vi "Command.vi"(7 "Cryo Idx":i32, 8 "error in (no error)":errorcluster, 9 "Options":string, 10 "Command":T1 items=["STATUS", "COOLER", "E", "ERROR", "KD", "KI", "KP", "LOGIN", "LOGOUT", "MODE", "P", "PWOUT", "SENSOR", "TC", "TEMP RJ", "TTARGET", "VERSION"], 11 "CryoCoolerAVC in":refnum<class "CryoCoolerAVC.lvclass">) -> (0 "error out":errorcluster, 2 "Response":string[](array[string]), 3 "CryoCoolerAVC out":refnum<class "CryoCoolerAVC.lvclass">)   [LabVIEW 2024, in "CryoCoolerAVC.lvclass"]
uses:
  CryoCoolerAVC.lvclass
  CryoCoolerAVC Command enum.ctl
  CryoCoolerAVC.lvclass/CryoCoolerAVC.ctl
  Cryo Cooler.lvclass
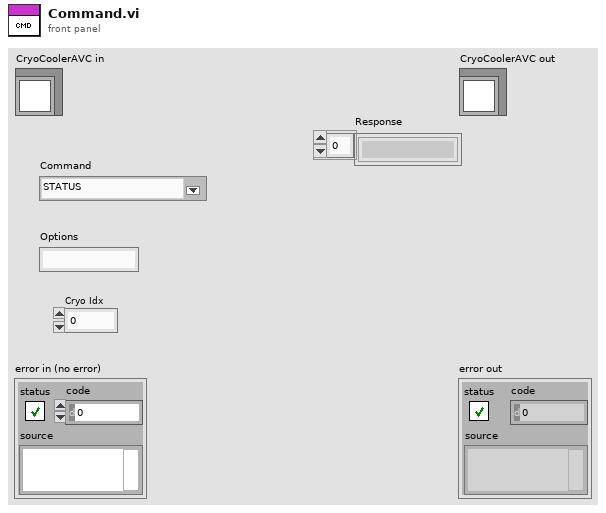
[diagram p1: front panel]
types:
  T1 = typedef "CryoCoolerAVC Command enum.ctl" = u16
  T2 = typedef "CryoCoolerAVC.lvclass/CryoCoolerAVC Settings.ctl" = cluster{"CryoTek 1 Addr":refnum<visa-resource-name>, "CryoTek 2 Addr":refnum<visa-resource-name>}
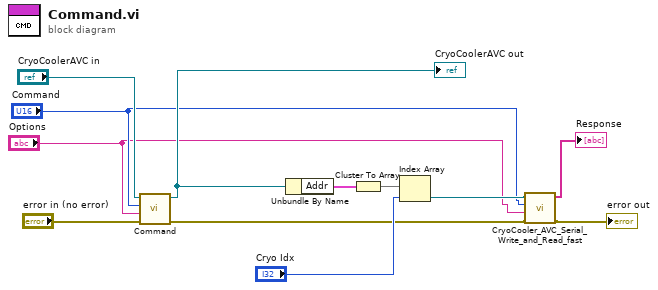
[diagram p0: block diagram]
diagram:
  n1 = call-parent "Command.vi"("error in (no error)"="error in (no error)", "Options"="Options", "Command"="Command", "Cryo Cooler in"="CryoCoolerAVC in") -> ("error out"=w6:errorcluster, "Cryo Cooler out"=w10:refnum<class "CryoCoolerAVC.lvclass">)  [unwired: 5 in, 1 out]
  "CryoCoolerAVC out" <- w10
  n2 = Unbundle By Name(w10) -> ("Addr"=w9:T2)
  n3 = Cluster To Array(cluster=w9) -> (array=w8:refnum<visa-resource-name>[])
  n4 = Index Array(array=w8, index="Cryo Idx") -> (element=w5:refnum<visa-resource-name>)
  n5 = call "CryoCooler_AVC_Serial_Write_and_Read_fast.vi"("error in (no error)"=w6, "Command Options"="Options", "Command"="Command", "VISA Resource (write)"=w5) -> ("error out"=→"error out":errorcluster, "read string array"=→"Response":string[])  [unwired: 5 in, 1 out]
